vi "Read Data.vi"(8 "error in":errorcluster, 11 "TCP in":refnum<class "TCP.lvclass">) -> (0 "error out":errorcluster, 2 "Data Read":string, 3 "TCP out":refnum<class "TCP.lvclass">)   [LabVIEW 2021, in "TCP.lvclass"]
uses:
  TCP.lvclass
  TCP.lvclass/TCP.ctl
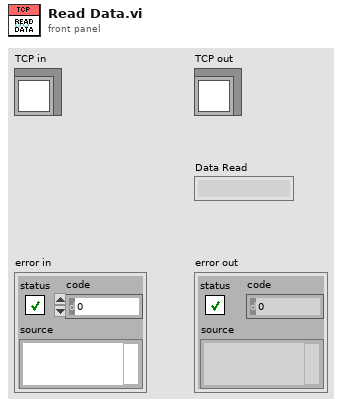
[diagram p1: front panel]
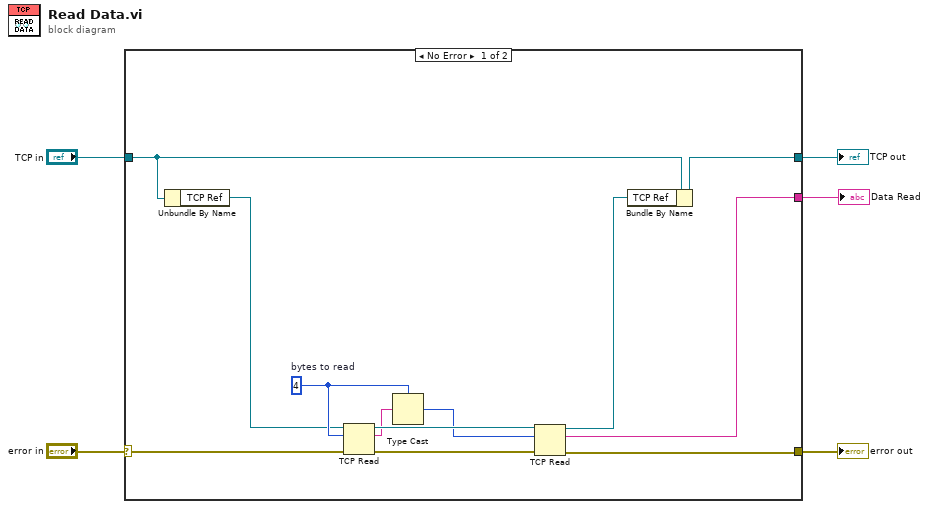
[diagram p0: block diagram]
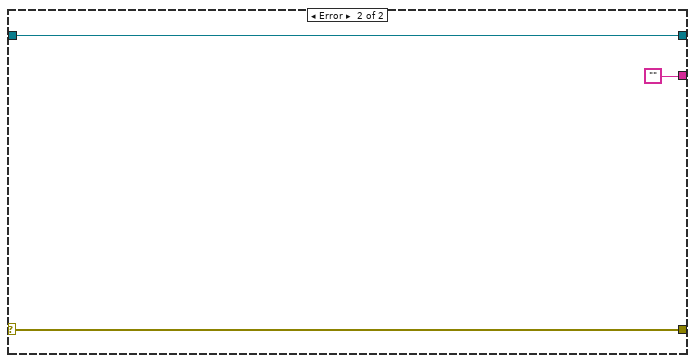
[diagram p2: hidden frame]
diagram:
  n1 = case shown="No Error" "error in" {
    selector: "error in" -> [w14 w19]
    tunnel: [w10 w19] -> w4
    tunnel: "TCP in" -> [w7 w20]
    tunnel: [w9 w20] -> w2
    tunnel: [w11 ""] -> w1
    frame No Error {
      w15 = 4  # bytes to read
      n2 = Unbundle By Name(w7) -> ("TCP Ref"=w6:refnum<k5>)
      n3 = TCP Read(connection ID=w6, bytes to read=w15, error in (no error)=w14) -> (connection ID out=w17:refnum<k5>, data out=w16:string, error out=w13:errorcluster)  [unwired: 2 in]
      n4 = Type Cast(type=w15, x=w16) -> (*(type *) &x=w12:i32)
      n5 = TCP Read(connection ID=w17, bytes to read=w12, error in (no error)=w13) -> (connection ID out=w8:refnum<k5>, data out=w11:string, error out=w10:errorcluster)  [unwired: 2 in]
      n6 = Bundle By Name(cluster=w7, "TCP Ref"=w8) -> (w9:refnum<class "TCP.lvclass">)
    }
    frame Error {
    }
  }
  "error out" <- w4
  "TCP out" <- w2
  "Data Read" <- w1
